vi "FindFaces.vi"() -> ()   [LabVIEW 2018]
panel:
  out "Image to process":picture
  out "Processed image":picture
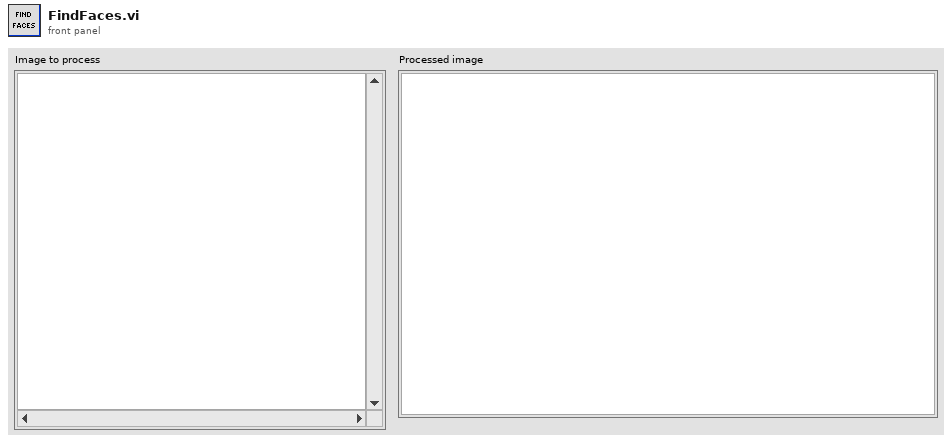
[diagram p1: front panel]
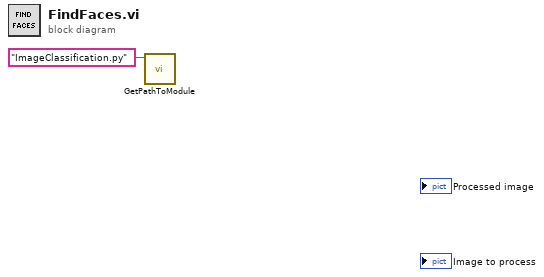
[diagram p0: block diagram]
diagram:
  n1 = call "GetPathToModule.vi"("module name"="ImageClassification.py") -> ()  [unwired: 10 in, 1 out]
